vi "motorMove.vi"(4 "position":dbl, 5 "Device in":refnum<k24>) -> (2 "Device out":refnum<k24>)   [LabVIEW 2014]
doc: "André Romero - 2017\nandretec@ifsc.usp.br"
uses:
  C:/UserLab/andre/GITs/andretec/Thorlabs-Vector-Move/kinesisTec/Kinesis/Thorlabs.MotionControl.TCube.DCServoCLI.dll
  Kinesis/Thorlabs.MotionControl.TCube.DCServoCLI.dll
  motorsGlobalVar.vi
panel:
  out "timeout i":i32
  out "Delay time":u32
  out "index of element":i32=2
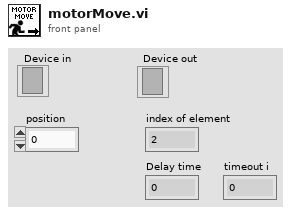
[diagram p1: front panel]
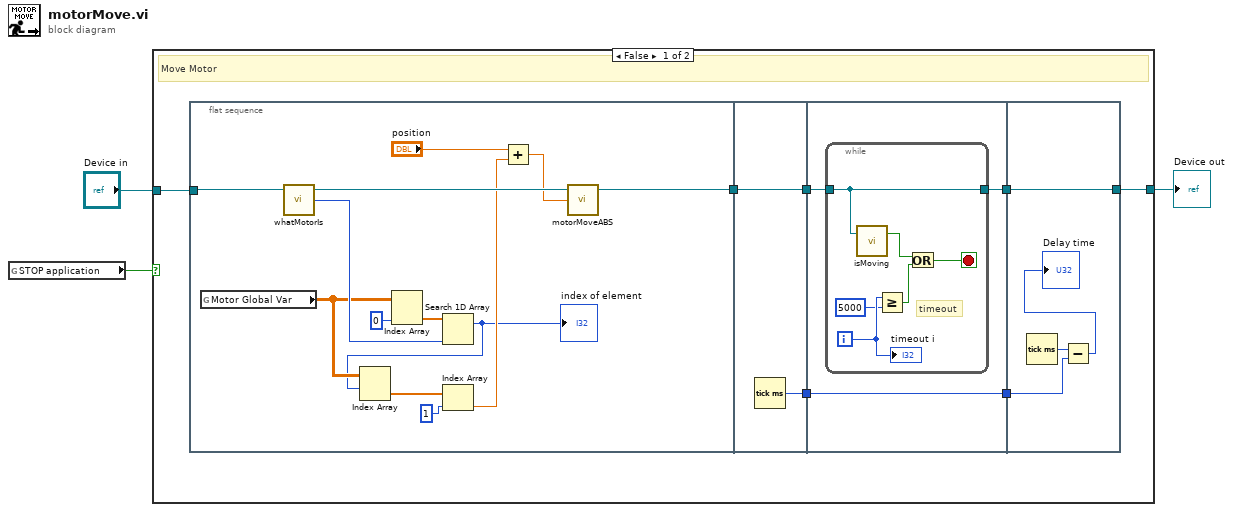
[diagram p0: block diagram]
diagram:
  n1 = global read "motorsGlobalVar.vi" "STOP application"() -> (w1:bool)
  n2 = case shown="False" w1 {
    tunnel: [w5 w39] -> w3
    tunnel: "Device in" -> [w4 w39]
    frame False {
      # "Move Motor"
      n3 = flat-sequence {
        tunnel: [w12] -> w10
        tunnel: w4 -> [w11]
        tunnel: w10 -> [w25]
        tunnel: [w25] -> w9
        tunnel: [w24] -> w8
        tunnel: w9 -> [w27]
        tunnel: [w28] -> w7
        tunnel: w8 -> [w26]
        tunnel: [w26] -> w6
        tunnel: [w38] -> w5
        tunnel: w7 -> [w38]
        tunnel: w6 -> [w36]
        frame #0 {
          n4 = global read "motorsGlobalVar.vi" "Motor Global Var"() -> (w16:dbl[][])
          n5 = call "whatMotorIs.vi"("Device in"=w11) -> ("SerialNumber"=w19:u32, "Device out"=w22:refnum<k24>)  [unwired: 3 in]
          n6 = Index Array(array=w16, index (col)=0 ("disabled index (col)")) -> (element=w20:dbl[])  [unwired: 1 in]
          n7 = Search 1D Array(1D array=w20, element=w19) -> (index of element=w13:i32)  [unwired: 1 in]
          "index of element" <- w13
          n8 = Index Array(array=w16, index (row)=w13) -> (element=w18:dbl[])  [unwired: 1 in]
          n9 = Index Array(array=w18, index=1) -> (element=w14:dbl)
          n10 = Add(x="position", y=w14) -> (x+y=w15:dbl)
          n11 = call "motorMoveABS.vi"("position"=w15, "Device in"=w22) -> ("Device out"=w12:refnum<k24>)  [unwired: 3 in]
        }
        frame #1 {
          n12 = Tick Count (ms)() -> (millisecond timer value=w24:u32)
        }
        frame #2 {
          n13 = while {
            tunnel: [w34] -> w28
            tunnel: w27 -> [w34]
            i -> [w32]
            stop <- w30 stop-if-true
            # "timeout"
            n14 = call "isMoving.vi"("Device in"=w34) -> ("IsMoving"=w33:bool)  [unwired: 2 in]
            n15 = Greater Or Equal?(x=w32, y=5000) -> (x >= y?=w29:bool)
            n16 = Or(x=w33, y=w29) -> (x .or. y?=w30:bool)
            "timeout i" <- w32
          }
        }
        frame #3 {
          n17 = Tick Count (ms)() -> (millisecond timer value=w37:u32)
          n18 = Subtract(x=w37, y=w36) -> (x-y=→"Delay time":u32)
        }
      }
    }
    frame True {
      # "if STOP is TRUE -> stop application"
    }
  }
  "Device out" <- w3
